vi "fgt get pressure Status.vi"(8 "error in (no error)":errorcluster, 11 "pressureIndex":u32) -> (0 "error out":errorcluster)   [LabVIEW 2020, in "fgt_SDK.lvlib"]
doc: "Get detailed information of pressure channel status. \nThis function is meant to be invoked after calling a pressure related function which returns an error code.\nRetrieved information of last error contains controller position and a string detail."
uses:
  fgt_SDK.lvlib
  TypeDefs/fgt_STATUS_INFO.ctl
  TypeDefs/fgt_INSTRUMENT_TYPE.ctl
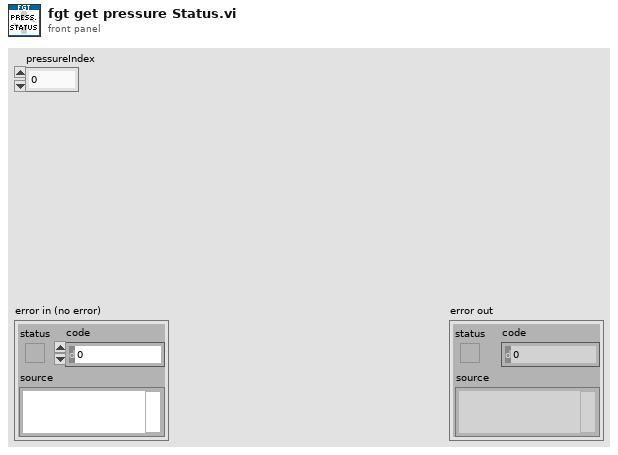
[diagram p1: front panel]
types:
  T1 = typedef "fgt_SDK.lvlib/fgt_STATUS_INFO.ctl" = cluster{"InstrType":T2, "instrSN":u16, "errorCode":u8, "infoCode":u8, "detail":string}
  T2 = typedef "fgt_SDK.lvlib/fgt_INSTRUMENT_TYPE.ctl" = enum32{"None", "MFCS", "MFCS_EZ", "FRP", "LineUP", "IPS"}
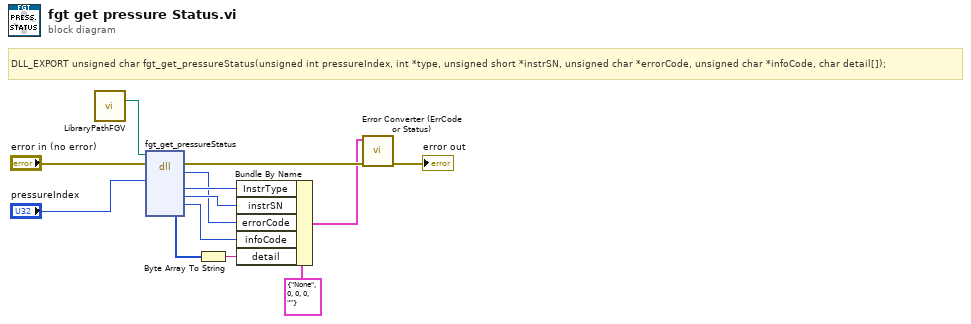
[diagram p0: block diagram]
diagram:
  # "DLL_EXPORT unsigned char fgt_get_pressureStatus(unsigned int pressureIndex, int *type, unsigned short *instrSN, unsigned char *errorCode, unsigned char *infoCode, char detail[]);"
  n1 = call "LibraryPathFGV.vi"() -> ("Path Out"=w1:path)  [unwired: 14 in, 1 out]
  n2 = dll-call lib="C:/Workspace/fgt-SDK/LabVIEW/dlls/fgt_SDK_*.*" fn="fgt_get_pressureStatus"(path in=w1, error in="error in (no error)", "pressureIndex"="pressureIndex") -> (error out=w11:errorcluster, "return type"=w4:u8, "type"=w8:i32, "instrSN"=w7:u16, "infoCode"=w6:u8, "detail"=w3:i8[])  [unwired: 6 in, 1 out]
  n3 = Byte Array To String(unsigned byte array=w3) -> (string=w2:string)
  n4 = Bundle By Name(cluster=T1 {"InstrType"=enum."None", "instrSN"=0, "errorCode"=0, "infoCode"=0, "detail"=""} ("Cluster"), "InstrType"=w8, "instrSN"=w7, "errorCode"=w4, "infoCode"=w6, "detail"=w2) -> (w5:T1)
  n5 = call "Error Converter (ErrCode or Status).vi"("error in (no error)"=w11, "StatusInfo"=w5) -> ("error out"=→"error out":errorcluster)  [unwired: 9 in]
